vi "String Check Output Result.vi"(9 "Output Value in":cluster{"Name":string, "Variant Data":variant}, 10 "Step Output in":T5, 11 "Execution in":refnum<data-value>) -> (2 "Measure Result out":T1, 3 "Execution out":refnum<data-value>)   [LabVIEW 2015, in "Execution.lvclass"]
uses:
  Execution.lvclass
  Step/STEP_OUTPUT.ctl
  Step/OUTPUT_DATA_TYPE.ctl
  OutputUI/OUTPUT_CHECK_TYPE.ctl
  Step/OUTPUT_VALUE_TYPE.ctl
  STEP_MEASURE_RESULT.ctl
  Step/STEP_STATUS.ctl
  <vilib>/Utility/error.llb/DialogType.ctl
  Get Limit Value String.vi
  <vilib>/regexp/Match Regular Expression.xnode
  Step.lvclass
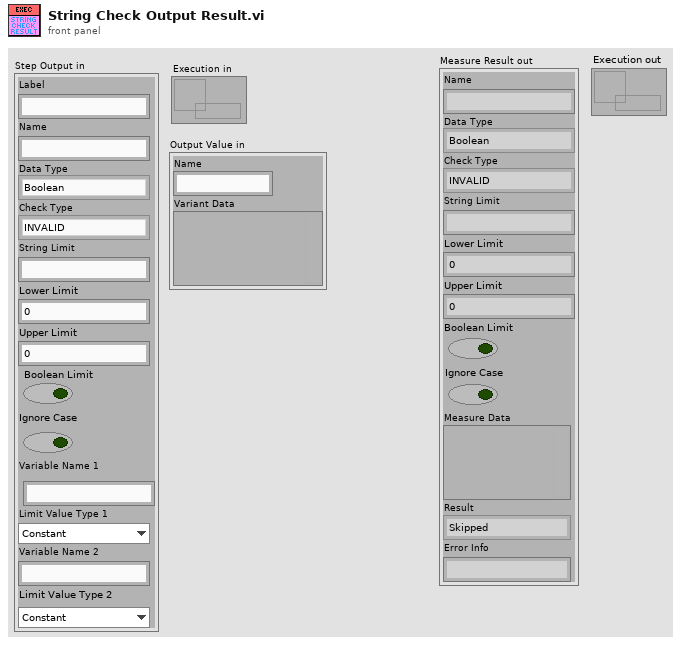
[diagram p1: front panel]
types:
  T1 = typedef "Execution.lvclass/STEP_MEASURE_RESULT.ctl" = cluster{"Name":string, "Data Type":T2, "Check Type":T3, "String Limit":string, "Lower Limit":dbl, "Upper Limit":dbl, "Boolean Limit":bool, "Ignore Case":bool, "Measure Data":variant, "Result":T4, "Error Info":string}
  T2 = typedef "Step.lvclass/OUTPUT_DATA_TYPE.ctl" = enum16{"Boolean", "String", "Numeric", "Other"}
  T3 = typedef "Step.lvclass/OUTPUT_CHECK_TYPE.ctl" = enum16{"INVALID", "DO_NOT_CHECK", "RECORD", "VARIABLE", "EQUAL", "NOT_EQUAL", "STR_CONTAINS", "STR_START_WITH", "STR_END_WITH", "STR_REGEX_MATCH", "NUM_GT", "NUM_LT", "NUM_GE", "NUM_LE", "NUM_RANGE", "NUM_RANGE_BDY"}
  T4 = typedef "Step.lvclass/STEP_STATUS.ctl" = enum16{"Skipped", "Done", "Passed", "Failed", "Error"}
  T5 = typedef "Step.lvclass/STEP_OUTPUT.ctl" = cluster{"Label":string, "Name":string, "Data Type":T2, "Check Type":T3, "String Limit":string, "Lower Limit":dbl, "Upper Limit":dbl, "Boolean Limit":bool, "Ignore Case":bool, "Variable Name 1":string, "Limit Value Type 1":T6, "Variable Name 2":string, "Limit Value Type 2":T6}
  T6 = typedef "Step.lvclass/OUTPUT_VALUE_TYPE.ctl" = enum16{"Constant", "Variable"}
  T7 = typedef "DialogType.ctl" = u16
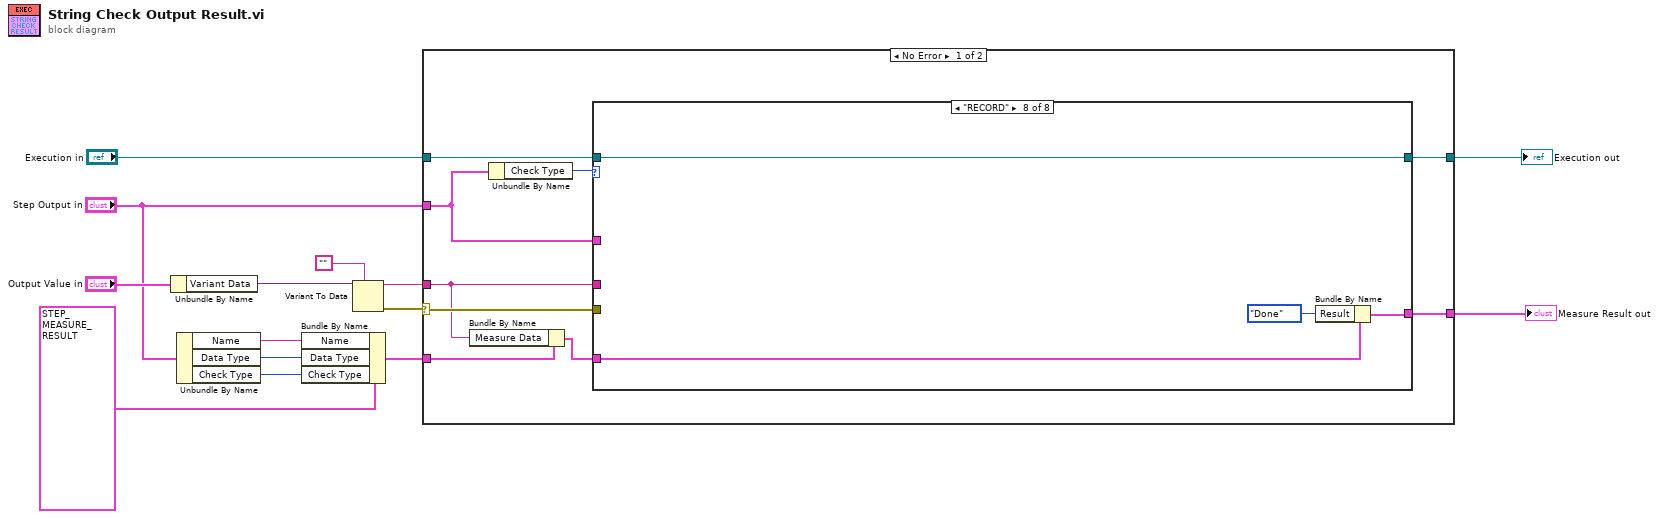
[diagram p0: block diagram]
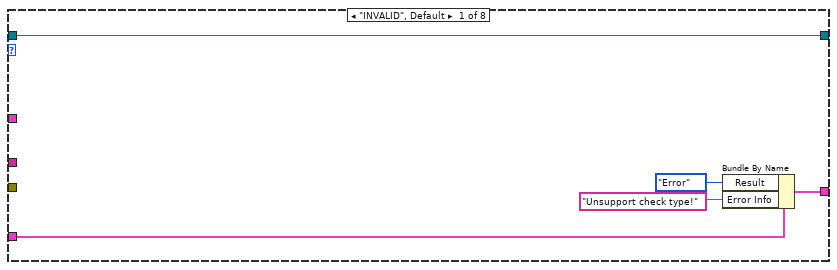
[diagram p2: hidden frame]
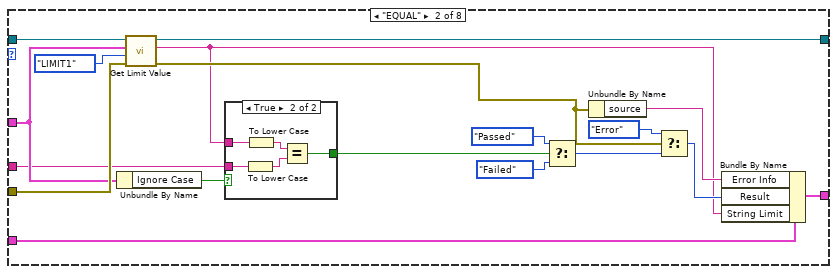
[diagram p3: hidden frame]
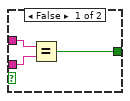
[diagram p4: hidden frame]
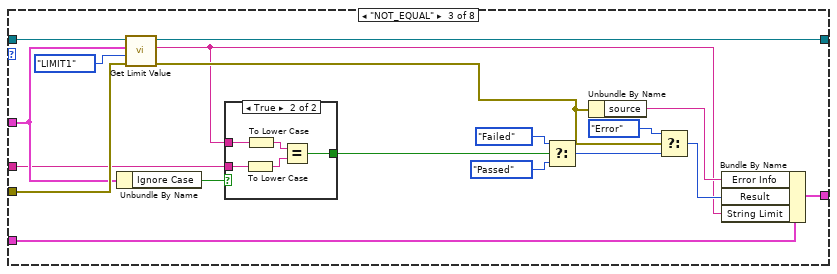
[diagram p5: hidden frame]
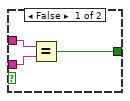
[diagram p6: hidden frame]
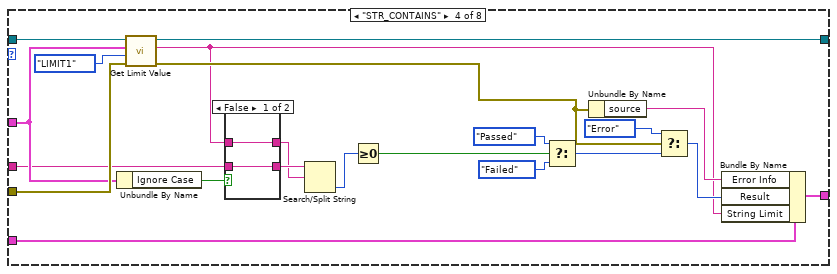
[diagram p7: hidden frame]
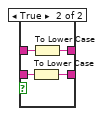
[diagram p8: hidden frame]
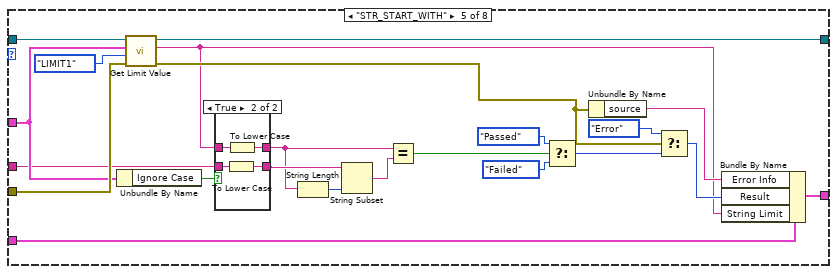
[diagram p9: hidden frame]
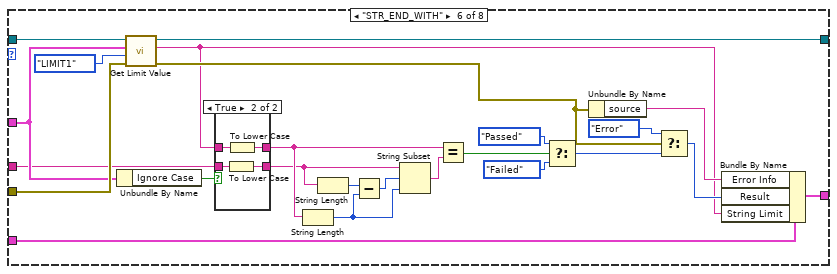
[diagram p11: hidden frame]
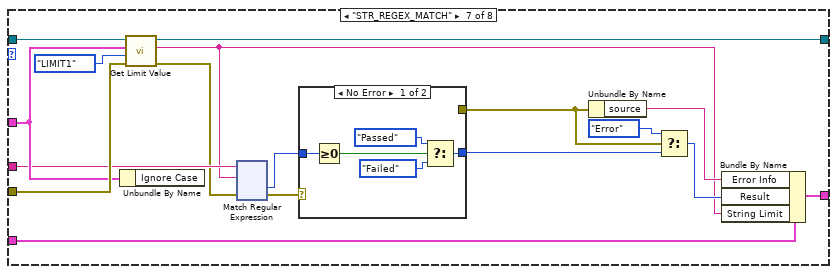
[diagram p13: hidden frame]
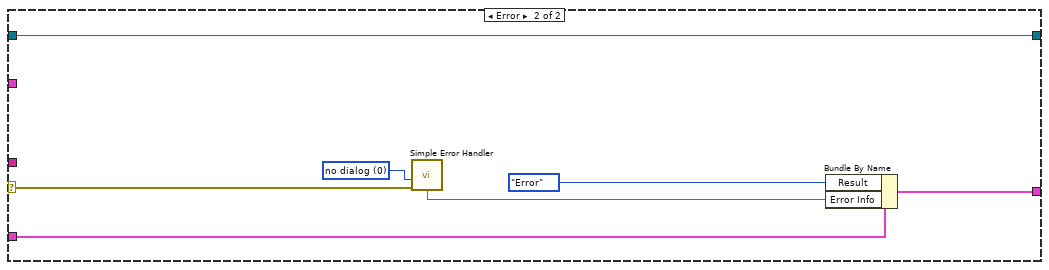
[diagram p15: hidden frame]
diagram:
  n1 = Unbundle By Name("Output Value in") -> ("Variant Data"=w12:variant)
  n2 = Unbundle By Name("Step Output in") -> ("Name"=w5:string, "Data Type"=w4:T2, "Check Type"=w3:T3)
  n3 = Bundle By Name(cluster=T1 {"Name"="", "Data Type"=enum."Boolean", "Check Type"=enum."INVALID", "String Limit"="", "Lower Limit"=0.0, "Upper Limit"=0.0, "Boolean Limit"=FALSE, "Ignore Case"=FALSE, "Measure Data"=variant, "Result"=enum."Skipped", "Error Info"=""} ("Measure Result"), "Name"=w5, "Data Type"=w4, "Check Type"=w3) -> (w2:T1)
  n4 = Variant To Data(type="", Variant=w12) -> (data=w10:string, error out=w14:errorcluster)  [unwired: 1 in]
  n5 = case shown="No Error" w14 {
    selector: w14 -> [w20 w312]
    tunnel: "Step Output in" -> [w23 _]
    tunnel: w10 -> [w18 _]
    tunnel: "Execution in" -> [w22 w311]
    tunnel: [w21 w311] -> w8
    tunnel: w2 -> [w19 w310]
    tunnel: [w16 w307] -> w1
    frame No Error {
      n6 = Bundle By Name(cluster=w19, "Measure Data"=w18) -> (w17:T1)
      n7 = Unbundle By Name(w23) -> ("Check Type"=w15:T3)
      n8 = case shown="\"RECORD\"" w15 {
        tunnel: w23 -> [_ w33 w59 w88 w116 w146 w173 _]
        tunnel: w18 -> [_ w31 w57 w86 w114 w144 w172 _]
        tunnel: w22 -> [w28 w38 w64 w93 w121 w151 w177 w303]
        tunnel: [w28 w37 w63 w92 w120 w150 w176 w303] -> w21
        tunnel: w20 -> [_ w36 w62 w91 w119 w149 w175 _]
        tunnel: w17 -> [w27 w42 w68 w97 w125 w155 w181 w306]
        tunnel: [w24 w39 w65 w94 w122 w152 w178 w305] -> w16
        frame "INVALID", Default {
          n9 = Bundle By Name(cluster=w27, "Result"=STEP_STATUS."Error" ("Status"), "Error Info"="Unsupport check type!") -> (w24:T1)
        }
        frame "EQUAL" {
          n10 = Unbundle By Name(w33) -> ("Ignore Case"=w32:bool)
          n11 = call-poly "Get Limit Value.vi"("error in (no error)"=w36, "Limit"=enum16{"LIMIT1", "LIMIT2"}."LIMIT1", "Step Output in"=w33, "Execution in"=w38) -> ("error out"=w34:errorcluster, "Limit Value"=w29:string, "Execution out"=w37:refnum<data-value>)  [unwired: 5 in]
          n12 = case shown="True" w32 {
            tunnel: w29 -> [w49 w54]
            tunnel: w31 -> [w48 w53]
            tunnel: [w47 w50] -> w30
            frame False {
              n13 = Equal?(x=w49, y=w48) -> (x = y?=w47:bool)
            }
            frame True {
              n14 = To Lower Case(string=w53) -> (all lower case string=w51:string)
              n15 = To Lower Case(string=w54) -> (all lower case string=w52:string)
              n16 = Equal?(x=w52, y=w51) -> (x = y?=w50:bool)
            }
          }
          n17 = Select(t=STEP_STATUS."Passed" ("Status"), s=w30, f=STEP_STATUS."Failed" ("Status")) -> (s? t:f=w44:T4)
          n18 = Unbundle By Name(w34) -> ("source"=w40:string)
          n19 = Select(t=STEP_STATUS."Error" ("Status"), s=w34, f=w44) -> (s? t:f=w41:T4)
          n20 = Bundle By Name(cluster=w42, "Error Info"=w40, "Result"=w41, "String Limit"=w29) -> (w39:T1)
        }
        frame "NOT_EQUAL" {
          n21 = Unbundle By Name(w59) -> ("Ignore Case"=w58:bool)
          n22 = call-poly "Get Limit Value.vi"("error in (no error)"=w62, "Limit"=enum16{"LIMIT1", "LIMIT2"}."LIMIT1", "Step Output in"=w59, "Execution in"=w64) -> ("error out"=w60:errorcluster, "Limit Value"=w55:string, "Execution out"=w63:refnum<data-value>)  [unwired: 5 in]
          n23 = case shown="True" w58 {
            tunnel: w55 -> [w75 w80]
            tunnel: w57 -> [w74 w79]
            tunnel: [w73 w76] -> w56
            frame False {
              n24 = Equal?(x=w75, y=w74) -> (x = y?=w73:bool)
            }
            frame True {
              n25 = To Lower Case(string=w79) -> (all lower case string=w77:string)
              n26 = To Lower Case(string=w80) -> (all lower case string=w78:string)
              n27 = Equal?(x=w78, y=w77) -> (x = y?=w76:bool)
            }
          }
          n28 = Select(t=STEP_STATUS."Failed" ("Status"), s=w56, f=STEP_STATUS."Passed" ("Status")) -> (s? t:f=w70:T4)
          n29 = Unbundle By Name(w60) -> ("source"=w66:string)
          n30 = Select(t=STEP_STATUS."Error" ("Status"), s=w60, f=w70) -> (s? t:f=w67:T4)
          n31 = Bundle By Name(cluster=w68, "Error Info"=w66, "Result"=w67, "String Limit"=w55) -> (w65:T1)
        }
        frame "STR_CONTAINS" {
          n32 = Unbundle By Name(w88) -> ("Ignore Case"=w87:bool)
          n33 = call-poly "Get Limit Value.vi"("error in (no error)"=w91, "Limit"=enum16{"LIMIT1", "LIMIT2"}."LIMIT1", "Step Output in"=w88, "Execution in"=w93) -> ("error out"=w89:errorcluster, "Limit Value"=w85:string, "Execution out"=w92:refnum<data-value>)  [unwired: 5 in]
          n34 = case shown="False" w87 {
            tunnel: w85 -> [w103 w107]
            tunnel: w86 -> [w102 w106]
            tunnel: [w103 w105] -> w83
            tunnel: [w102 w104] -> w84
            frame False {
            }
            frame True {
              n35 = To Lower Case(string=w106) -> (all lower case string=w104:string)
              n36 = To Lower Case(string=w107) -> (all lower case string=w105:string)
            }
          }
          n37 = Search/Split String(string=w84, search string/char (-)=w83) -> (offset of match=w82:i32)  [unwired: 1 in, 2 out]
          n38 = Greater Or Equal To 0?(x=w82) -> (x >= 0?=w81:bool)
          n39 = Select(t=STEP_STATUS."Passed" ("Status"), s=w81, f=STEP_STATUS."Failed" ("Status")) -> (s? t:f=w99:T4)
          n40 = Unbundle By Name(w89) -> ("source"=w95:string)
          n41 = Select(t=STEP_STATUS."Error" ("Status"), s=w89, f=w99) -> (s? t:f=w96:T4)
          n42 = Bundle By Name(cluster=w97, "Error Info"=w95, "Result"=w96, "String Limit"=w85) -> (w94:T1)
        }
        frame "STR_START_WITH" {
          n43 = Unbundle By Name(w116) -> ("Ignore Case"=w115:bool)
          n44 = call-poly "Get Limit Value.vi"("error in (no error)"=w119, "Limit"=enum16{"LIMIT1", "LIMIT2"}."LIMIT1", "Step Output in"=w116, "Execution in"=w121) -> ("error out"=w117:errorcluster, "Limit Value"=w113:string, "Execution out"=w120:refnum<data-value>)  [unwired: 5 in]
          n45 = case shown="True" w115 {
            tunnel: w113 -> [w131 w135]
            tunnel: w114 -> [w130 w134]
            tunnel: [w131 w133] -> w109
            tunnel: [w130 w132] -> w110
            frame False {
            }
            frame True {
              n46 = To Lower Case(string=w134) -> (all lower case string=w132:string)
              n47 = To Lower Case(string=w135) -> (all lower case string=w133:string)
            }
          }
          n48 = String Length(string=w109) -> (length=w111:i32)
          n49 = String Subset(string=w110, length (rest)=w111) -> (substring=w112:string)  [unwired: 1 in]
          n50 = Equal?(x=w109, y=w112) -> (x = y?=w108:bool)
          n51 = Select(t=STEP_STATUS."Passed" ("Status"), s=w108, f=STEP_STATUS."Failed" ("Status")) -> (s? t:f=w127:T4)
          n52 = Unbundle By Name(w117) -> ("source"=w123:string)
          n53 = Select(t=STEP_STATUS."Error" ("Status"), s=w117, f=w127) -> (s? t:f=w124:T4)
          n54 = Bundle By Name(cluster=w125, "Error Info"=w123, "Result"=w124, "String Limit"=w113) -> (w122:T1)
        }
        frame "STR_END_WITH" {
          n55 = Unbundle By Name(w146) -> ("Ignore Case"=w145:bool)
          n56 = call-poly "Get Limit Value.vi"("error in (no error)"=w149, "Limit"=enum16{"LIMIT1", "LIMIT2"}."LIMIT1", "Step Output in"=w146, "Execution in"=w151) -> ("error out"=w147:errorcluster, "Limit Value"=w143:string, "Execution out"=w150:refnum<data-value>)  [unwired: 5 in]
          n57 = case shown="True" w145 {
            tunnel: w143 -> [w161 w165]
            tunnel: w144 -> [w160 w164]
            tunnel: [w161 w163] -> w138
            tunnel: [w160 w162] -> w137
            frame False {
            }
            frame True {
              n58 = To Lower Case(string=w164) -> (all lower case string=w162:string)
              n59 = To Lower Case(string=w165) -> (all lower case string=w163:string)
            }
          }
          n60 = String Length(string=w138) -> (length=w141:i32)
          n61 = String Length(string=w137) -> (length=w140:i32)
          n62 = Subtract(x=w140, y=w141) -> (x-y=w142:i32)
          n63 = String Subset(string=w137, offset (0)=w142, length (rest)=w141) -> (substring=w139:string)
          n64 = Equal?(x=w138, y=w139) -> (x = y?=w136:bool)
          n65 = Select(t=STEP_STATUS."Passed" ("Status"), s=w136, f=STEP_STATUS."Failed" ("Status")) -> (s? t:f=w157:T4)
          n66 = Unbundle By Name(w147) -> ("source"=w153:string)
          n67 = Select(t=STEP_STATUS."Error" ("Status"), s=w147, f=w157) -> (s? t:f=w154:T4)
          n68 = Bundle By Name(cluster=w155, "Error Info"=w153, "Result"=w154, "String Limit"=w143) -> (w152:T1)
        }
        frame "STR_REGEX_MATCH" {
          n69 = Unbundle By Name(w173) -> ()  [unwired: 1 out]
          n70 = call-poly "Get Limit Value.vi"("error in (no error)"=w175, "Limit"=enum16{"LIMIT1", "LIMIT2"}."LIMIT1", "Step Output in"=w173, "Execution in"=w177) -> ("error out"=w170:errorcluster, "Limit Value"=w171:string, "Execution out"=w176:refnum<data-value>)  [unwired: 5 in]
          n71 = xnode "Match Regular Expression"("input string"=w172, "regular expression"=w171, "error in"=w170) -> ("offset past match"=w168:i32, "error out"=w169:errorcluster)  [unwired: 3 in, 3 out]
          n72 = case shown="No Error" w169 {
            selector: w169 -> [_ w188]
            tunnel: w168 -> [w184 _]
            tunnel: [w183 _] -> w167
            tunnel: [_ w188] -> w166
            frame No Error {
              n73 = Greater Or Equal To 0?(x=w184) -> (x >= 0?=w185:bool)
              n74 = Select(t=STEP_STATUS."Passed" ("Status"), s=w185, f=STEP_STATUS."Failed" ("Status")) -> (s? t:f=w183:T4)
            }
            frame Error {
            }
          }
          n75 = Unbundle By Name(w166) -> ("source"=w179:string)
          n76 = Select(t=STEP_STATUS."Error" ("Status"), s=w166, f=w167) -> (s? t:f=w180:T4)
          n77 = Bundle By Name(cluster=w181, "Error Info"=w179, "Result"=w180, "String Limit"=w171) -> (w178:T1)
        }
        frame "RECORD" {
          n78 = Bundle By Name(cluster=w306, "Result"=STEP_STATUS."Done") -> (w305:T1)
        }
      }
    }
    frame Error {
      w313 = T7 0 items=["no dialog", "OK message", "continue or stop message", "OK message + warnings", "continue/stop + warnings"] ("type of dialog (OK msg:1)")
      n79 = call <vilib>:"Simple Error Handler.vi"("type of dialog (OK msg:1)"=w313, "error in (no error)"=w312) -> ("message"=w309:string)  [unwired: 3 in, 4 out]
      n80 = Bundle By Name(cluster=w310, "Result"=STEP_STATUS."Error" ("Status"), "Error Info"=w309) -> (w307:T1)
    }
  }
  "Execution out" <- w8
  "Measure Result out" <- w1
